vi "TapeWaitForTapeMonitorCam.vi"(10 "MinTapeMonMax":dbl format="%#_13g", 11 "TapeDrive in":refnum<class "TapeDrive.lvclass">) -> (1 "maxCounts":dbl[](graph), 3 "TapeDrive out":refnum<class "TapeDrive.lvclass">)   [LabVIEW 2020, in "TapeDrive.lvclass"]
uses:
  TapeDrive.lvclass
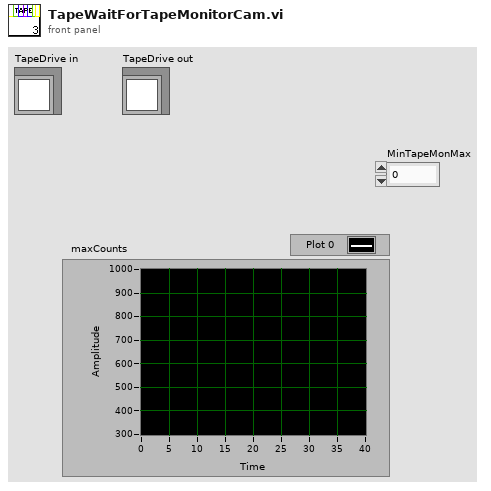
[diagram p1: front panel]
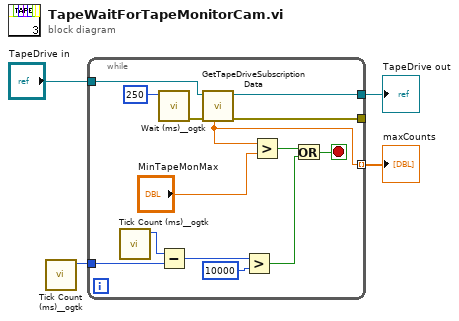
[diagram p0: block diagram]
diagram:
  n1 = call <userlib>:"Tick Count (ms)__ogtk.vi"() -> ("millisecond timer value"=w1:u32)  [unwired: 10 in, 1 out]
  n2 = while {
    tunnel: "TapeDrive in" -> [w18]
    tunnel: [w17] -> w3
    tunnel: [w13] -> w4 mode=indexing
    tunnel: [w14] -> _
    tunnel: w1 -> [w9]
    stop <- w5 stop-if-true
    n3 = call <userlib>:"Tick Count (ms)__ogtk.vi"() -> ("millisecond timer value"=w10:u32)  [unwired: 10 in, 1 out]
    n4 = call <userlib>:"Wait (ms)__ogtk.vi"("milliseconds to wait"=u32 250) -> ("error out"=w16:errorcluster)  [unwired: 9 in, 1 out]
    n5 = Subtract(x=w10, y=w9) -> (x-y=w8:u32)
    n6 = call "GetTapeDriveSubscriptionData.vi"("error in (no error)"=w16, "TapeDrive in"=w18) -> ("error out"=w14:errorcluster, "TapeDrive in 2"=w17:refnum<class "TapeDrive.lvclass">, "TapeMonMaxCounts"=w13:dbl)  [unwired: 3 in, 4 out]
    n7 = Greater?(x=w8, y=u32 10000) -> (0:w6:bool)
    n8 = Greater?(x=w13, y="MinTapeMonMax") -> (0:w11:bool)
    n9 = Or(x=w11, y=w6) -> (x .or. y?=w5:bool)
  }
  "maxCounts" <- w4
  "TapeDrive out" <- w3
